vi "Read Config Record.vi"(8 "error in (no error)":errorcluster, 10 "Record":T1, 11 "Elevator Controller Actor in":refnum<class "Elevator Controller Actor.lvclass">) -> (0 "error out":errorcluster, 3 "Elevator Controller Actor out":refnum<class "Elevator Controller Actor.lvclass">)   [LabVIEW 2019]
uses:
  Configuration Database Actor/Configuration Database Actor/Record -Cluster.ctl
  Configuration Database Actor/Configuration Database Actor/Configuration Database Actor.lvclass
  Elevator Controller Actor.lvclass
  C:/Program Files (x86)/National Instruments/LabVIEW 2019/vi.lib/ActorFramework/Actor/Actor.lvclass
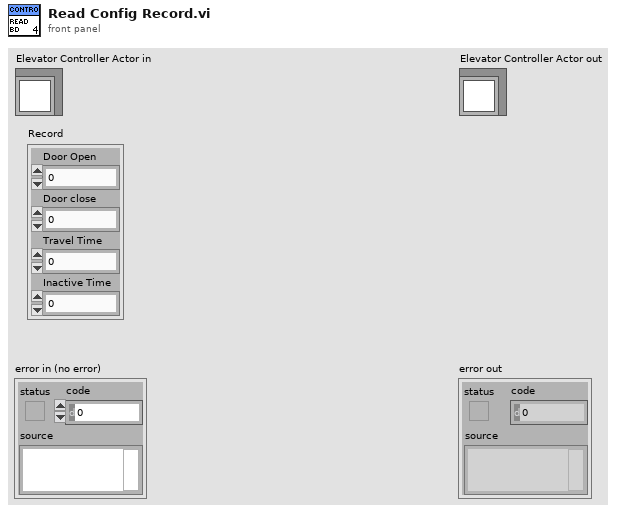
[diagram p1: front panel]
types:
  T1 = typedef "Configuration Database Actor.lvlib/Configuration Database Actor.lvclass/Record -Cluster.ctl" = cluster{"Door Open":dbl, "Door close":dbl, "Travel Time":dbl, "Inactive Time":dbl}
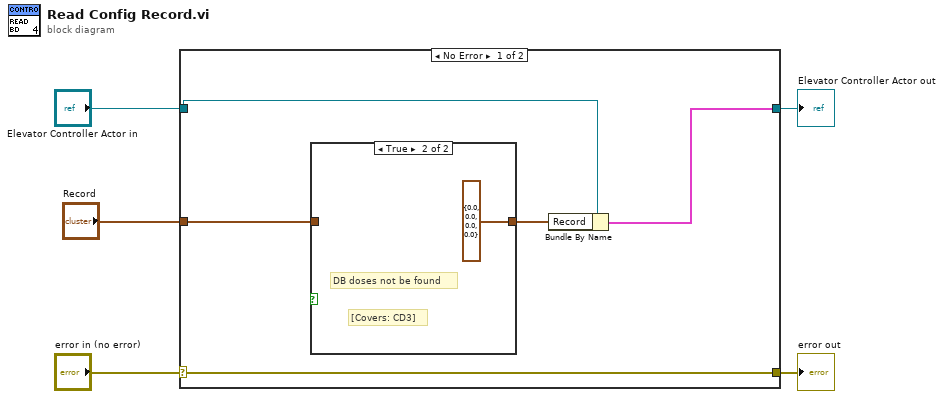
[diagram p0: block diagram]
diagram:
  n1 = case shown="No Error" "error in (no error)" {
    selector: "error in (no error)" -> [w10 w14]
    tunnel: [w10 w14] -> w4
    tunnel: [w8 w13] -> w2
    tunnel: "Elevator Controller Actor in" -> [w9 w13]
    tunnel: "Record" -> [w7 _]
    frame No Error {
      n2 = case shown="True" {
        selector: _ -> [_ _]
        tunnel: [w11 T1 {"Door Open"=0.0, "Door close"=0.0, "Travel Time"=0.0, "Inactive Time"=0.0} ("Record")] -> w6
        tunnel: w7 -> [w11 _]
        frame False {
        }
        frame True {
          # "[Covers: CD3]"
          # "DB doses not be found"
        }
      }
      n3 = Bundle By Name(cluster=w9, "Record"=w6) -> (w8:cluster{})
    }
    frame Error {
    }
  }
  "error out" <- w4
  "Elevator Controller Actor out" <- w2
